vi "Remove Session.vi"(8 "error in (no error)":errorcluster, 11 "Session in":refnum<class "Session.lvclass">) -> (0 "error out":errorcluster, 3 "Session out":refnum<class "Session.lvclass">)   [LabVIEW 2020, in "HTTP Server.lvlib" / "Session.lvclass"]
uses:
  Session.lvclass
  Session.lvclass/Session.ctl
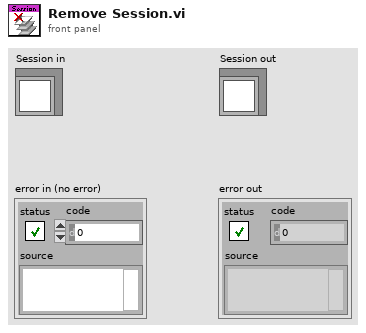
[diagram p1: front panel]
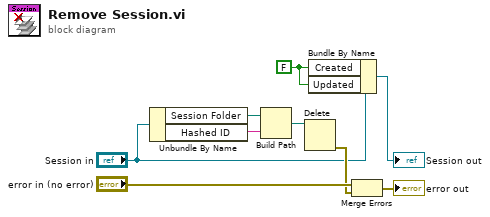
[diagram p0: block diagram]
diagram:
  w1 = FALSE ("Created")
  n1 = Unbundle By Name("Session in") -> ("Session Folder"=w8:path, "Hashed ID"=w7:string)
  n2 = Build Path(base path=w8, name or relative path=w7) -> (appended path=w6:path)
  n3 = Delete(path (use dialog)=w6) -> (error out=w4:errorcluster)  [unwired: 4 in, 2 out]
  n4 = Bundle By Name(cluster="Session in", "Created"=w1, "Updated"=w1) -> (→"Session out":refnum<class "Session.lvclass">)
  n5 = Merge Errors("error in (no error)", w4) -> (→"error out":errorcluster)
